vi "trash_Update Configuration Command.vi"(8 "error in":errorcluster, 10 "Config JSON":string, 11 "CoreOOB_Rx in":refnum<class "ChanMngOOB_Rx.lvclass">) -> (0 "error out":errorcluster, 3 "CoreOOB_Rx out":refnum<class "ChanMngOOB_Rx.lvclass">)   [LabVIEW 2021]
uses:
  ChanMngOOB_Rx.lvclass/ChanMngOOB_Rx.ctl
  <vilib>/CIF Foundation/CIF Out of Band Commands/CIFOutOfBand.lvclass
  Typedef/OOB ChnMng Commands.ctl
  ChanMngOOB_Rx.lvclass
  <vilib>/addons/_JKI.lib/Serialization/JSON/JKI JSON Serialization.lvlib
  Typedef/Template Payload.ctl
  Typedef/Channel Connection Data.ctl
  Typedef/Channel Fault Data.ctl
  C:/Program Files/National Instruments/LabVIEW 2021/vi.lib/CIF Foundation/CIF Out of Band Commands/CIFOutOfBand.lvclass
  <vilib>/CIF Foundation/CIF Out of Band Commands/Typedef/OOB Container.ctl
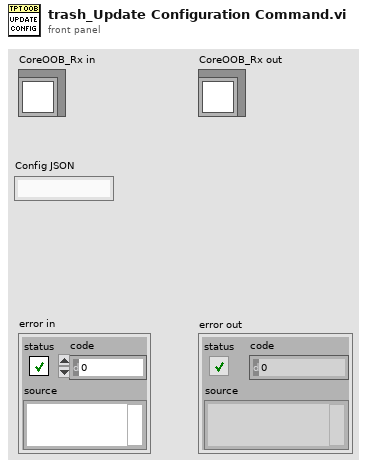
[diagram p1: front panel]
types:
  T1 = typedef "CIFOutOfBand.lvclass/OOB Container.ctl" = cluster{"Commands (bitwise)":u64, "Payload":variant}
  T2 = typedef "ChanMngOOB_Rx.lvclass/OOB ChnMng Commands.ctl" = enum8{"Start", "Pause", "Stop", "RefreshStats", "UpdateConfig", "Connect Channel", "Force Channel", "Update Clock Map"}
  T3 = typedef "ChanMngOOB_Rx.lvclass/Template Payload.ctl" = cluster{"Connections":T4[], "Forces":T5[]}
  T4 = typedef "ChanMngOOB_Rx.lvclass/Channel Connection Data.ctl" = cluster{"Publisher Name":string, "Subscriber Name":string, "Connection Data":u8[]}
  T5 = typedef "ChanMngOOB_Rx.lvclass/Channel Fault Data.ctl" = cluster{"Channel Name":string, "Force Data":u8[], "Force Active":bool}
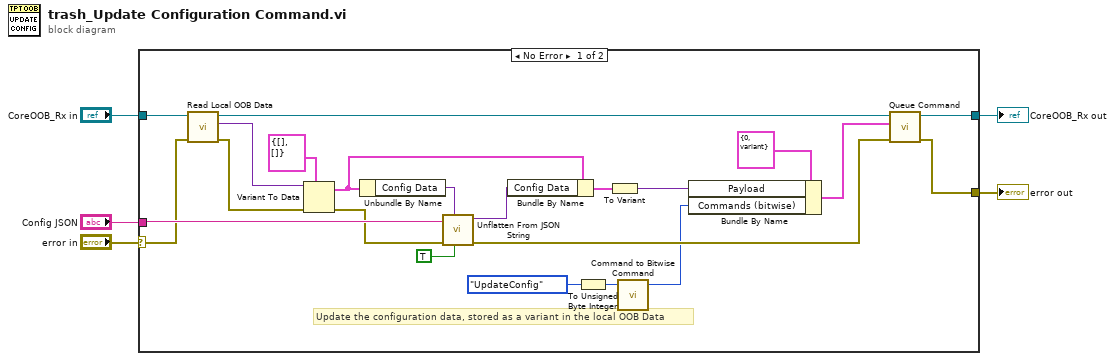
[diagram p0: block diagram]
diagram:
  n1 = case shown="No Error" "error in" {
    selector: "error in" -> [w21 w29]
    tunnel: [w26 w29] -> w4
    tunnel: "CoreOOB_Rx in" -> [w22 w28]
    tunnel: [w27 w28] -> w2
    tunnel: "Config JSON" -> [w25 _]
    frame No Error {
      # "Update the configuration data, stored as a variant in the local OOB Data"
      n2 = call <vilib>:"Read Local OOB Data.vi"("error in"=w21, "OOB in"=w22) -> ("error out"=w16:errorcluster, "Local OOB Data"=w20:variant, "OOB out"=w10:refnum<class "ChanMngOOB_Rx.lvclass">)  [unwired: 7 in]
      n3 = Variant To Data(error in=w16, type=T3 {"Connections"=[], "Forces"=[]} ("Template Payload"), Variant=w20) -> (data=w17:T3, error out=w15:errorcluster)
      n4 = Unbundle By Name(w17) -> ("Config Data"=w18:variant)
      n5 = call <vilib>:"Unflatten From JSON String.vi"("Nulls as Defaults (F)"=TRUE, "Type and Defaults"=w18, "error in (no error)"=w15, "JSON String"=w25) -> ("error out"=w11:errorcluster, "Variant"=w24:variant)  [unwired: 6 in]
      n6 = Bundle By Name(cluster=w17, "Config Data"=w24) -> (w12:T3)
      n7 = To Unsigned Byte Integer(number=OOB_ChnMng_Commands."UpdateConfig" ("OOB Main Commands")) -> (unsigned 8bit integer=w14:u8)
      n8 = To Variant(anything=w12) -> (Variant=w8:variant)
      n9 = call <vilib>:"Command to Bitwise Command.vi"("Command"=w14) -> ("bit command"=w7:u64)  [unwired: 3 in]
      n10 = Bundle By Name(cluster=T1 {"Commands (bitwise)"=0, "Payload"=variant} ("OOB Data"), "Payload"=w8, "Commands (bitwise)"=w7) -> (w6:T1)
      n11 = call <vilib>:"Queue Command.vi"("error in"=w11, "OOB Data"=w6, "OOB in"=w10) -> ("error out"=w26:errorcluster, "OOB out"=w27:refnum<class "ChanMngOOB_Rx.lvclass">)  [unwired: 7 in]
    }
    frame Error {
    }
  }
  "error out" <- w4
  "CoreOOB_Rx out" <- w2
